vi "Program Device.vi"(0 "Data Cluster In":T1={"Message"="", "Homed?"=FALSE, "NextState"=enum."Timeout", "G.Load"=0.0, "G.Position"=0.0, "Load#"=0, "[G.Loads]"=[], "[TotalLoads]"=[], "[Errors]"=[], "ZeroWait"=0, "Results"=[], "DwellWait"=FALSE, "Test Result"=FALSE, "[CondyleLoads]"=[], "[Max]"=[], "[Min]"=[], "Valid String?"=FALSE, "ScanTime"=timestamp(0 s since 1904-01-01), "ScannedString"="", "LabelDevID"=0, "MfgDate"=timestamp(0 s since 1904-01-01), "[EEPROM Cmds]"=[], "[CalData]"=[], "[A/Ds]"=[], "[A/Dmax]"=[], "[A/Dmin]"=[], "BattMax"=0.0, "BattMin"=0.0, "DwellTime"=2000, "PendingDeviceType"="", "Zero G.load"=0.0, "GAINC Value"="", "Programming Step"=enum."Load EEPROM", "Front Panel Program?"=FALSE, "Final Program?"=FALSE, "PCB Score"=100, "AssyScore"=100, "Pass/Fail #"="", "Result String"="", "Programming Mode"=enum."Initial Program", "Angle Test Step"=enum."Initialize", "Accel Values"=[], "Shutdown Counter"=0, "V1"=0, "V2"=0, "V3"=0, "V4"=0, "EEPROM Data"=[], "Counter"=0, "Page#"=0, "Timer"=timestamp(0 s since 1904-01-01), "Use Mark10?"=FALSE, "Eng-Result#"=0, "DUT Serial #"=0, "Scroll Message?"=FALSE, "Clear Message"=FALSE, "Batt Test Step "=enum."Initialize", "RXTX Window Found?"=FALSE, "Shutdown First Call?"=FALSE, "A2 Delay (msec)"=500, "Support Script"={"Script #"="", "Script Revision"="", "[OEMs]"=[], "[[DeviceTypes]]"=[], "[[DeviceTypesVals]]"=[], "[[List of Errors]]"=[], "Default GAINC"="", "[[ASICtrims]]"=[], "ID For Echo"="", "Condyle A CalFactor"=100, "Condyle B CalFactor"=100, "[OEMs Prefix]"=[], "Packet ID 18"="", "[[Force Table Load Test]]"=[], "[[Force Table AccurTest]]"=[]}, "Serial Table"={"Serial File Path"=path "", "[[Serial Lookup Table]]"=[], "Serial Device Info"=[], "Valid Serial?"=FALSE}, "Target Information"={"Target Brand"="", "Target DeviceType"="", "Target Serial#"=100, "Target Lot#"=0, "Target DevID"=0, "Target Channel"=5}, "Operator"="", "COM Port"="", "Config Path"=path "", "Tx Array"=[], "DUT Parameters"={"Channel"=0, "DeviceID"=0, "Script Rev"=0, "Month"=0, "Day"=0, "Year"=0, "Lot#"=0, "V1"=0, "V2"=0, "V3"=0, "V4"=0, "MFG"=0, "Cal FactorA 10"=0, "Cal FactorB 10  "=0, "Cal FactorA 16"=0, "Cal FactorB 16"=0, "ASICtrim"=[], "TmpChan"=0, "GAINC"="", "Brand"="", "Device"="", "Serial #"=0, "Batt310"=0, "Batt 280"=0}, "FTS Main?"=FALSE, "Loading"={"[Forces]"=[], "[Dwell]"=[], "Loading Step"=enum."Initialize Test"}, "Software Version"="", "Correction Factor"="", "Second Load Test"=FALSE, "Acc Loads"=[], "Mark10 Config"={"H2S%"=[80.0, 85.0, 90.0, 95.0, 100.0], "H2S Speed"=[12.0, 8.0, 6.0, 4.0, 2.0], "H to S"=2.0, "Home Speed"=1.0, "LoadWin"=0.0, "Load Speed"=0.0, "PID"={"Kp"=0.04, "Kd"=0.005001, "Ki"=2.9999999999999923e-05}}, "Channels"={"Transceiver Ch"=5, "Operating Ch"=5, "Start Ch"=0}, "Channel EEPROM"=[], "Load Notes"=[], "Engr Log?"=FALSE, "Time"=[], "Program Retry"=FALSE, "Operator Channel"="", "Target Channel "="", "New Data Program"=FALSE, "NFHU Pass?"=FALSE, "Cycle Number"=0, "Cal Cycle#"=0, "[Avg G.Loads] "=[], "[Avg A/Ds] "=[], "Cal Retry?"=FALSE, "[Total A/Ds]  "=[], "Cycle Num LA"=0, "LA Cycle# "=0, "Shim Num"=0, "Shim#  "=0, "Angle Test?"=FALSE} {"Mark10 Config"."PID"."Ki" min=0.0 max=200.0 format="%.6f"; "Mark10 Config"."PID"."Kd" min=0.0 max=200.0 format="%.6f"; "Mark10 Config"."PID"."Kp" min=0.0 max=200.0 format="%.6f"; "DUT Parameters"."ASICtrim" format="%02x"}, 11 "error in (no error)":errorcluster) -> (4 "Data Cluster Out":T1={"Message"="", "Homed?"=FALSE, "NextState"=enum."Timeout", "G.Load"=0.0, "G.Position"=0.0, "Load#"=0, "[G.Loads]"=[], "[TotalLoads]"=[], "[Errors]"=[], "ZeroWait"=0, "Results"=[], "DwellWait"=FALSE, "Test Result"=FALSE, "[CondyleLoads]"=[], "[Max]"=[], "[Min]"=[], "Valid String?"=FALSE, "ScanTime"=timestamp(0 s since 1904-01-01), "ScannedString"="", "LabelDevID"=0, "MfgDate"=timestamp(0 s since 1904-01-01), "[EEPROM Cmds]"=[], "[CalData]"=[], "[A/Ds]"=[], "[A/Dmax]"=[], "[A/Dmin]"=[], "BattMax"=0.0, "BattMin"=0.0, "DwellTime"=2000, "PendingDeviceType"="", "Zero G.load"=0.0, "GAINC Value"="", "Programming Step"=enum."Load EEPROM", "Front Panel Program?"=FALSE, "Final Program?"=FALSE, "PCB Score"=100, "AssyScore"=100, "Pass/Fail #"="", "Result String"="", "Programming Mode"=enum."Initial Program", "Angle Test Step"=enum."Initialize", "Accel Values"=[], "Shutdown Counter"=0, "V1"=0, "V2"=0, "V3"=0, "V4"=0, "EEPROM Data"=[], "Counter"=0, "Page#"=0, "Timer"=timestamp(0 s since 1904-01-01), "Use Mark10?"=FALSE, "Eng-Result#"=0, "DUT Serial #"=0, "Scroll Message?"=FALSE, "Clear Message"=FALSE, "Batt Test Step "=enum."Initialize", "RXTX Window Found?"=FALSE, "Shutdown First Call?"=FALSE, "A2 Delay (msec)"=500, "Support Script"={"Script #"="", "Script Revision"="", "[OEMs]"=[], "[[DeviceTypes]]"=[], "[[DeviceTypesVals]]"=[], "[[List of Errors]]"=[], "Default GAINC"="", "[[ASICtrims]]"=[], "ID For Echo"="", "Condyle A CalFactor"=100, "Condyle B CalFactor"=100, "[OEMs Prefix]"=[], "Packet ID 18"="", "[[Force Table Load Test]]"=[], "[[Force Table AccurTest]]"=[]}, "Serial Table"={"Serial File Path"=path "", "[[Serial Lookup Table]]"=[], "Serial Device Info"=[], "Valid Serial?"=FALSE}, "Target Information"={"Target Brand"="", "Target DeviceType"="", "Target Serial#"=100, "Target Lot#"=0, "Target DevID"=0, "Target Channel"=5}, "Operator"="", "COM Port"="", "Config Path"=path "", "Tx Array"=[], "DUT Parameters"={"Channel"=0, "DeviceID"=0, "Script Rev"=0, "Month"=0, "Day"=0, "Year"=0, "Lot#"=0, "V1"=0, "V2"=0, "V3"=0, "V4"=0, "MFG"=0, "Cal FactorA 10"=0, "Cal FactorB 10  "=0, "Cal FactorA 16"=0, "Cal FactorB 16"=0, "ASICtrim"=[], "TmpChan"=0, "GAINC"="", "Brand"="", "Device"="", "Serial #"=0, "Batt310"=0, "Batt 280"=0}, "FTS Main?"=FALSE, "Loading"={"[Forces]"=[], "[Dwell]"=[], "Loading Step"=enum."Initialize Test"}, "Software Version"="", "Correction Factor"="", "Second Load Test"=FALSE, "Acc Loads"=[], "Mark10 Config"={"H2S%"=[80.0, 85.0, 90.0, 95.0, 100.0], "H2S Speed"=[12.0, 8.0, 6.0, 4.0, 2.0], "H to S"=2.0, "Home Speed"=1.0, "LoadWin"=0.0, "Load Speed"=0.0, "PID"={"Kp"=0.04, "Kd"=0.005001, "Ki"=2.9999999999999923e-05}}, "Channels"={"Transceiver Ch"=5, "Operating Ch"=5, "Start Ch"=0}, "Channel EEPROM"=[], "Load Notes"=[], "Engr Log?"=FALSE, "Time"=[], "Program Retry"=FALSE, "Operator Channel"="", "Target Channel "="", "New Data Program"=FALSE, "NFHU Pass?"=FALSE, "Cycle Number"=0, "Cal Cycle#"=0, "[Avg G.Loads] "=[], "[Avg A/Ds] "=[], "Cal Retry?"=FALSE, "[Total A/Ds]  "=[], "Cycle Num LA"=0, "LA Cycle# "=0, "Shim Num"=0, "Shim#  "=0, "Angle Test?"=FALSE} {"Mark10 Config"."PID"."Ki" min=0.0 max=200.0 format="%.6f"; "Mark10 Config"."PID"."Kd" min=0.0 max=200.0 format="%.6f"; "Mark10 Config"."PID"."Kp" min=0.0 max=200.0 format="%.6f"; "DUT Parameters"."ASICtrim" format="%02x"}, 6 "Program Successful":bool, 15 "error out":errorcluster)   [LabVIEW 2015]
uses:
  Controls/LocalVars.ctl
  Controls/Gen2 FT states.ctl
  Controls/Iniial Device Programming.ctl
  ProgramStageControl.ctl
  Controls/Batt Cap Steps.ctl
  Controls/Support Script.ctl
  Controls/Serial Table.ctl
  Controls/Device Information.ctl
  Controls/InfoPacket.ctl
  Controls/Loading.ctl
  Controls/Load Step.ctl
  Controls/Mark10 Config.ctl
  Controls/PID parameters.ctl
  Controls/Channels.ctl
  RxTx/XceiverStates.ctl
  RxTx/XceiverCmds.ctl
  Controls/Gen2 FT Globals.vi
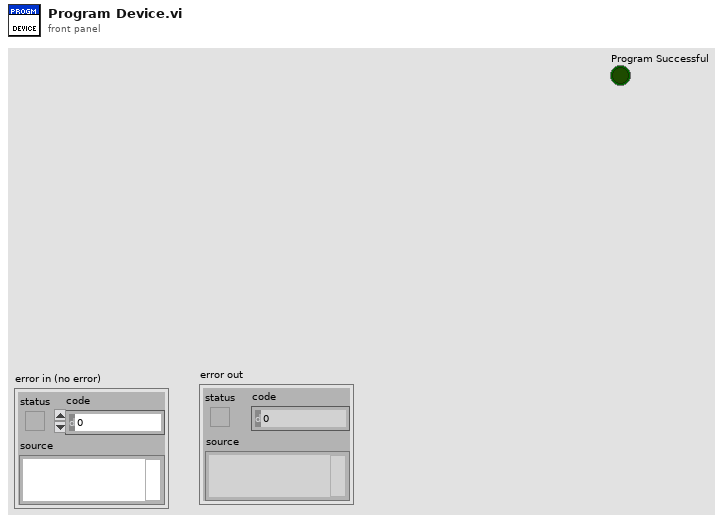
[diagram p1: front panel]
types:
  T1 = typedef "LocalVars.ctl" = cluster{"Message":string, "Homed?":bool, "NextState":T2, "G.Load":dbl, "G.Position":dbl, "Load#":i32, "[G.Loads]":dbl[], "[TotalLoads]":dbl[], "[Errors]":dbl[][], "ZeroWait":u32, "Results":dbl[], "DwellWait":bool, "Test Result":bool, "[CondyleLoads]":dbl[][], "[Max]":dbl[], "[Min]":dbl[], "Valid String?":bool, "ScanTime":timestamp, "ScannedString":string, "LabelDevID":u32, "MfgDate":timestamp, "[EEPROM Cmds]":u8[][], "[CalData]":u8[][], "[A/Ds]":dbl[][], "[A/Dmax]":dbl[], "[A/Dmin]":dbl[], "BattMax":dbl, "BattMin":dbl, "DwellTime":i32, "PendingDeviceType":string, "Zero G.load":dbl, "GAINC Value":string, "Programming Step":T3, "Front Panel Program?":bool, "Final Program?":bool, "PCB Score":i32, "AssyScore":i32, "Pass/Fail #":string, "Result String":string, "Programming Mode":T4, "Angle Test Step":enum16{"Initialize", "Get X", "Get Y", "Get Z", "Next Test"}, "Accel Values":dbl[][], "Shutdown Counter":u32, "V1":i32, "V2":i32, "V3":i32, "V4":i32, "EEPROM Data":i32[][], "Counter":i32, "Page#":i32, "Timer":timestamp, "Use Mark10?":bool, "Eng-Result#":u32, "DUT Serial #":i32, "Scroll Message?":bool, "Clear Message":bool, "Batt Test Step ":T5, "RXTX Window Found?":bool, "Shutdown First Call?":bool, "A2 Delay (msec)":i16, "Support Script":T6, "Serial Table":T7, "Target Information":T8, "Operator":string, "COM Port":string, "Config Path":path, "Tx Array":u8[], "DUT Parameters":T9, "FTS Main?":bool, "Loading":T10, "Software Version":string, "Correction Factor":string, "Second Load Test":bool, "Acc Loads":dbl[][], "Mark10 Config":T12, "Channels":T14, "Channel EEPROM":i32[][], "Load Notes":string[], "Engr Log?":bool, "Time":timestamp[], "Program Retry":bool, "Operator Channel":string, "Target Channel ":string, "New Data Program":bool, "NFHU Pass?":bool, "Cycle Number":i32, "Cal Cycle#":i32, "[Avg G.Loads] ":dbl[], "[Avg A/Ds] ":dbl[][], "Cal Retry?":bool, "[Total A/Ds]  ":dbl[][], "Cycle Num LA":i32, "LA Cycle# ":i32, "Shim Num":i32, "Shim#  ":i32, "Angle Test?":bool}
  T2 = typedef "Gen2 FT states.ctl" = enum16{"---------SETUP-------", "Initialization", "Read Support Data", "Initialize Mark-10", "Initialize Transceiver", "------UTILITIES------", "Change DUT Channel", "Find RxTx Window", "Reset Device", "Scan Channels", "Read Serial Lookup", "Shutdown Device", "ESTOP", "--------USER---------", "Timeout", "-----PROGRAM-----", "Program Device", "------MARK10--------", "Go Home", "MoveUp", "MoveDown", "Goto Load", "Goto Position", "Stop Motor", "---------TESTS--------", "Start Test", "Angle Test", "Load Test", "Load Accuracy Test", "Battery Test", "------RESULTS-------", "End Test", "Display Result", "--------EXIT--------", "Exit"}
  T3 = typedef "Iniial Device Programming.ctl" = enum16{"Load EEPROM", "Send First A1", "Send EEPROM", "Send A1", "Check EEPROM Echo", "Verify transmission", "Programming Successful", "Programming Failed"}
  T4 = typedef "ProgramStageControl.ctl" = enum16{"Initial Program", "GainC", "Scales"}
  T5 = typedef "Batt Cap Steps.ctl" = enum16{"Initialize", "Collect 2.8 Volts", "Collect 3.1 Volts", "Check Results"}
  T6 = typedef "Support Script.ctl" = cluster{"Script #":string, "Script Revision":string, "[OEMs]":string[], "[[DeviceTypes]]":string[][], "[[DeviceTypesVals]]":u16[][], "[[List of Errors]]":string[][], "Default GAINC":string, "[[ASICtrims]]":u8[][], "ID For Echo":string, "Condyle A CalFactor":i32, "Condyle B CalFactor":i32, "[OEMs Prefix]":string[], "Packet ID 18":string, "[[Force Table Load Test]]":dbl[][], "[[Force Table AccurTest]]":dbl[][]}
  T7 = typedef "Serial Table.ctl" = cluster{"Serial File Path":path, "[[Serial Lookup Table]]":string[][], "Serial Device Info":string[], "Valid Serial?":bool}
  T8 = typedef "Device Information.ctl" = cluster{"Target Brand":string, "Target DeviceType":string, "Target Serial#":i32, "Target Lot#":u32, "Target DevID":u32, "Target Channel":u8}
  T9 = typedef "InfoPacket.ctl" = cluster{"Channel":u8, "DeviceID":u32, "Script Rev":u8, "Month":u8, "Day":u8, "Year":u8, "Lot#":u32, "V1":u16, "V2":u16, "V3":u16, "V4":u16, "MFG":u8, "Cal FactorA 10":u8, "Cal FactorB 10  ":u8, "Cal FactorA 16":u8, "Cal FactorB 16":u8, "ASICtrim":u8[], "TmpChan":u8, "GAINC":string, "Brand":string, "Device":string, "Serial #":u64, "Batt310":u16, "Batt 280":u16}
  T10 = typedef "Loading.ctl" = cluster{"[Forces]":dbl[], "[Dwell]":dbl[], "Loading Step":T11}
  T11 = typedef "Load Step.ctl" = enum16{"Initialize Test", "Go Home", "Detect Dev Surface", "Wait to zero Device", "Zero Device", "Do Test", "Test Result"}
  T12 = typedef "Mark10 Config.ctl" = cluster{"H2S%":dbl[], "H2S Speed":dbl[], "H to S":dbl, "Home Speed":dbl, "LoadWin":dbl, "Load Speed":dbl, "PID":T13}
  T13 = typedef "PID parameters.ctl" = cluster{"Kp":dbl, "Kd":dbl, "Ki":dbl}
  T14 = typedef "Channels.ctl" = cluster{"Transceiver Ch":u8, "Operating Ch":u8, "Start Ch":u8}
  T15 = typedef "XceiverStates.ctl" = enum16{"Initialize", "Rx", "Tx", "Raw Mode", "Clear Buffer", "ClearEcho", "Read Buffer", "Close"}
  T16 = typedef "XceiverCmds.ctl" = enum8{"Get Window", "Set Window", "Load&Xmit", "Find Window", "Load CC1101", "Blink LED1", "Blink LED2", "Gen2 Mode", "Request Rev", "Gen2 Mode & Req Rev", "Load Device Settings", "Reset Xceiver", "Set Channel", "Read Channel"}
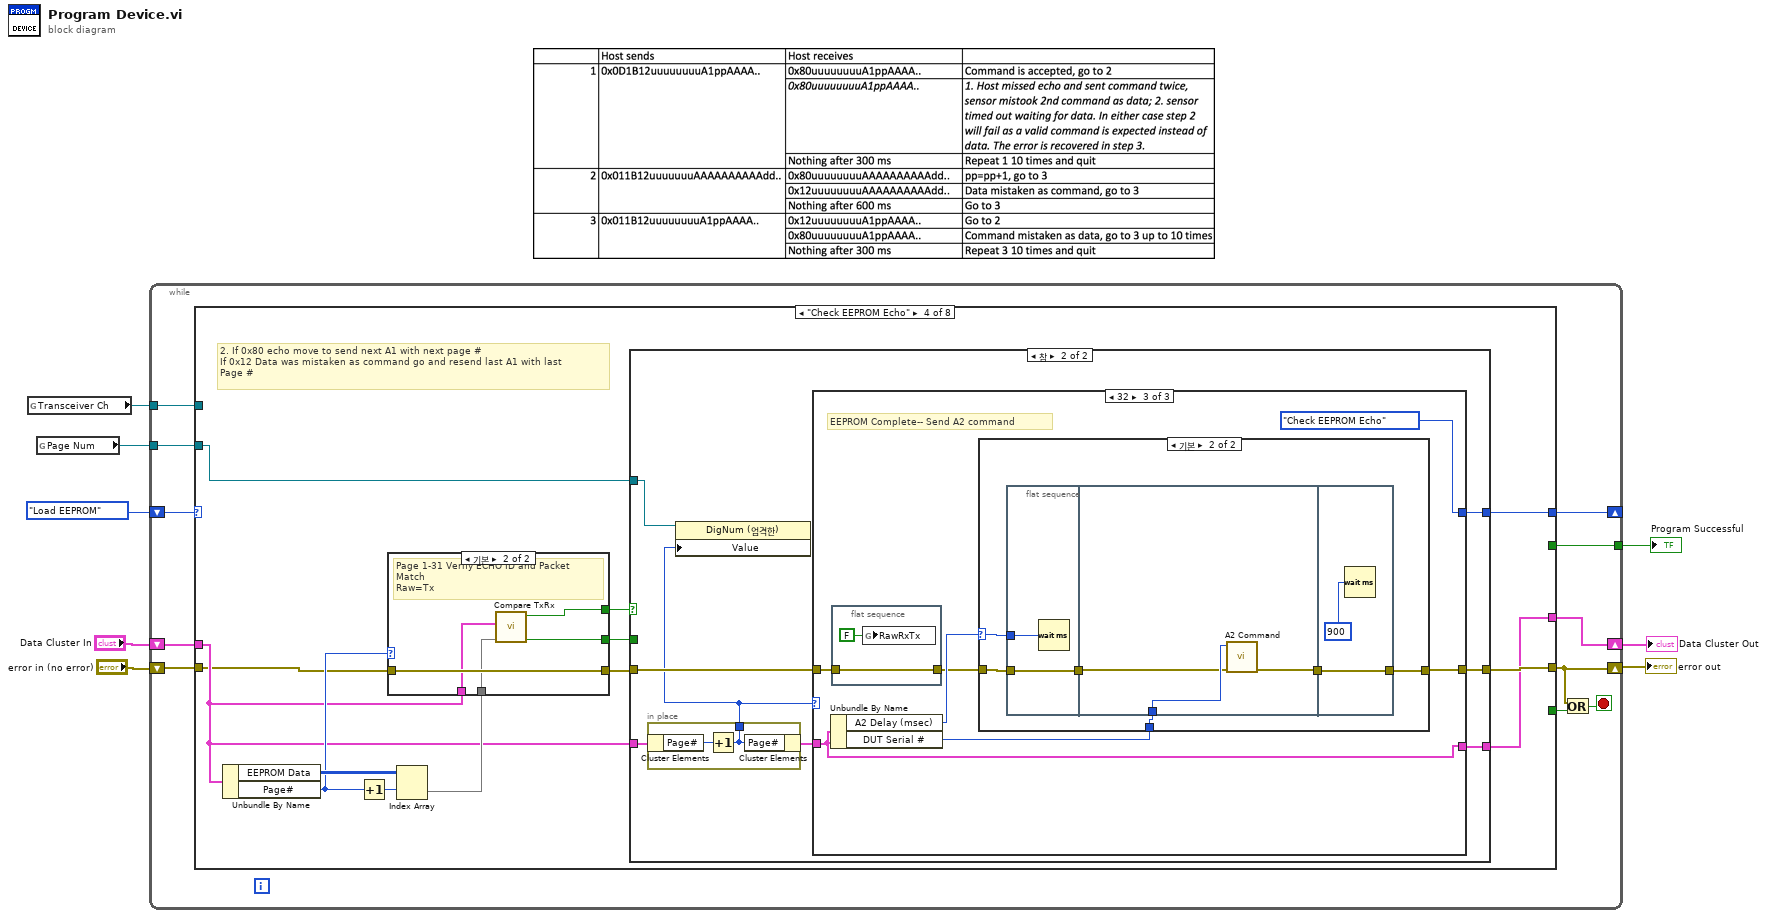
[diagram p0: block diagram]
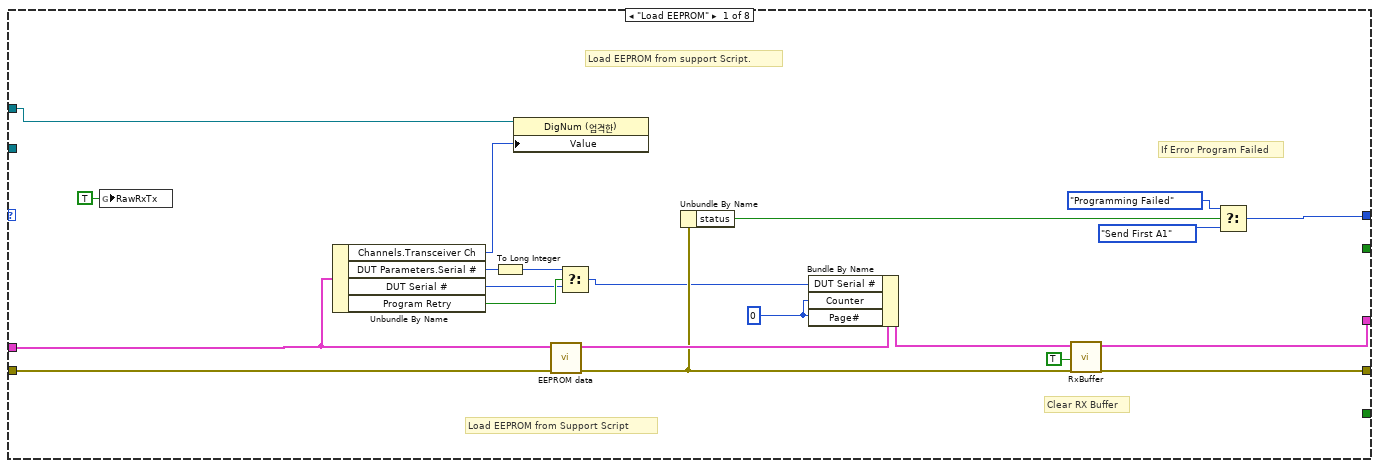
[diagram p2: hidden frame]
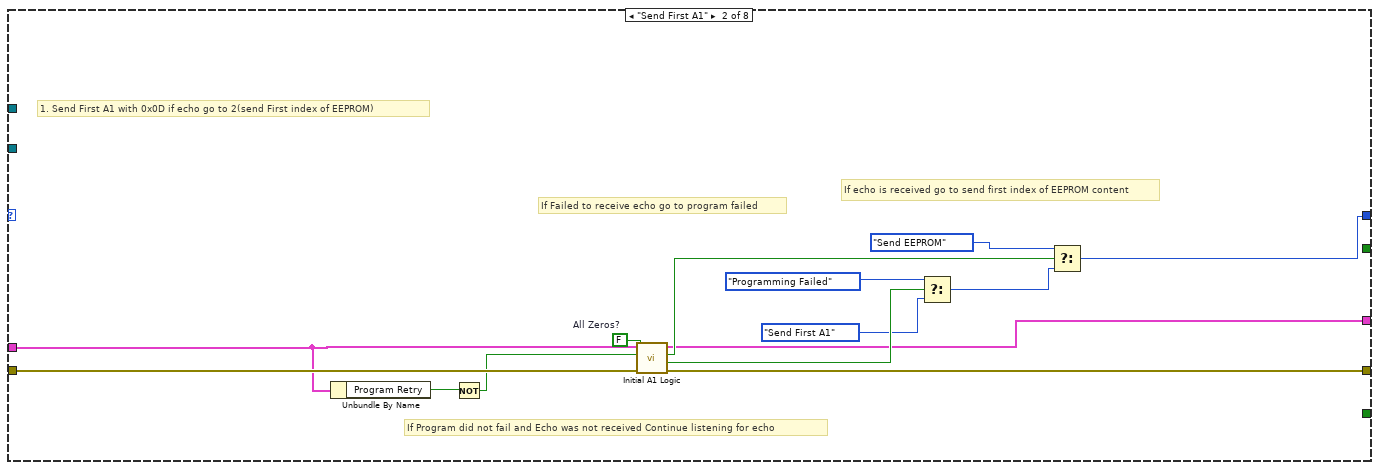
[diagram p3: hidden frame]
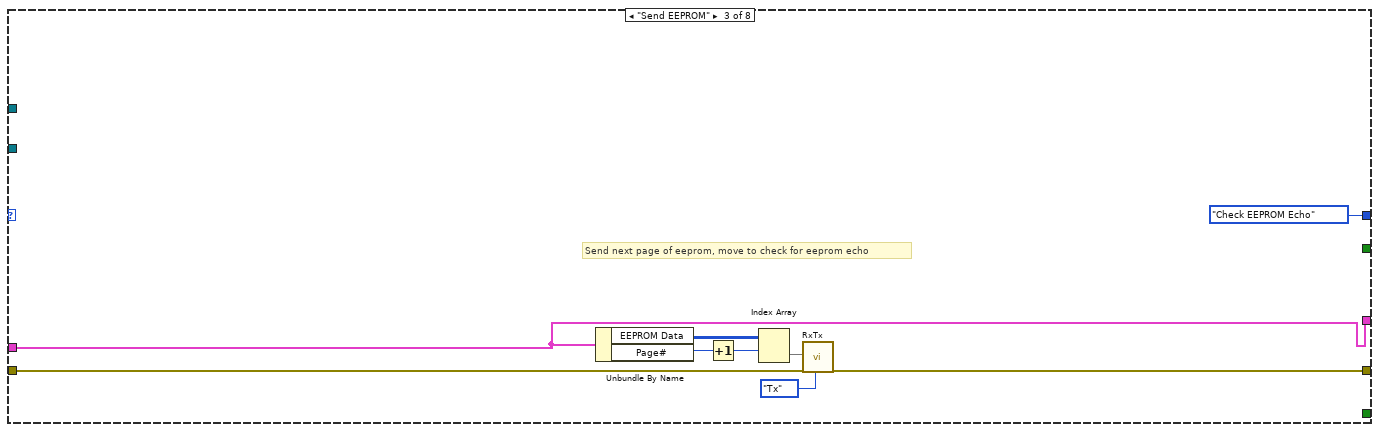
[diagram p4: hidden frame]
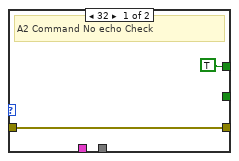
[diagram p5: hidden frame]
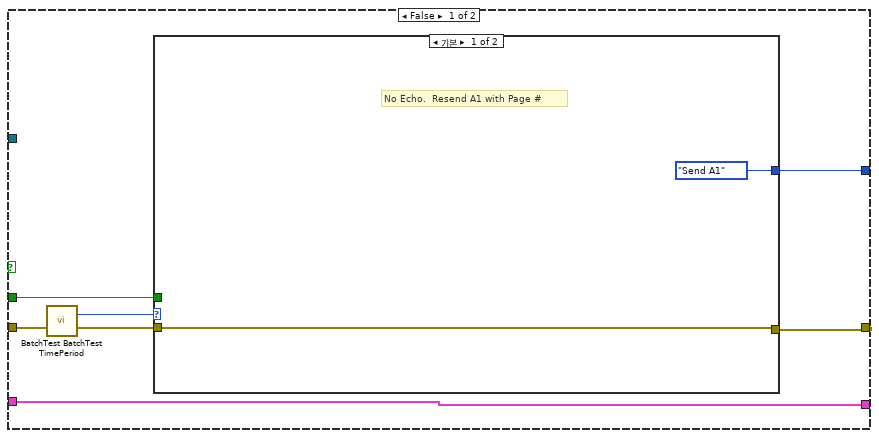
[diagram p6: hidden frame]
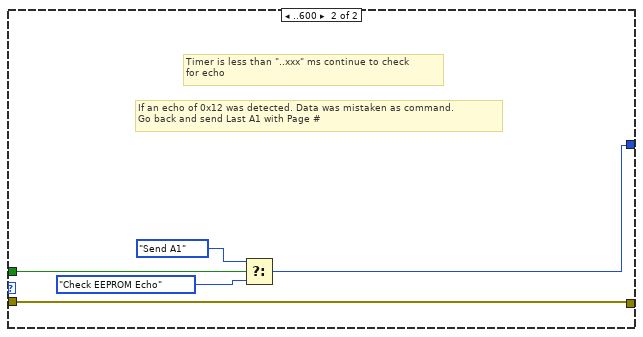
[diagram p7: hidden frame]
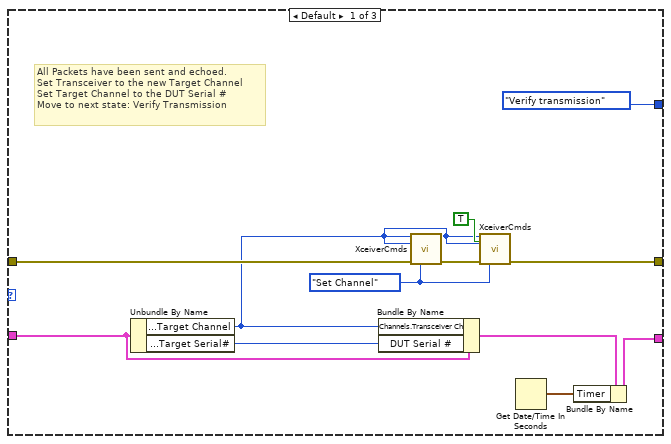
[diagram p8: hidden frame]
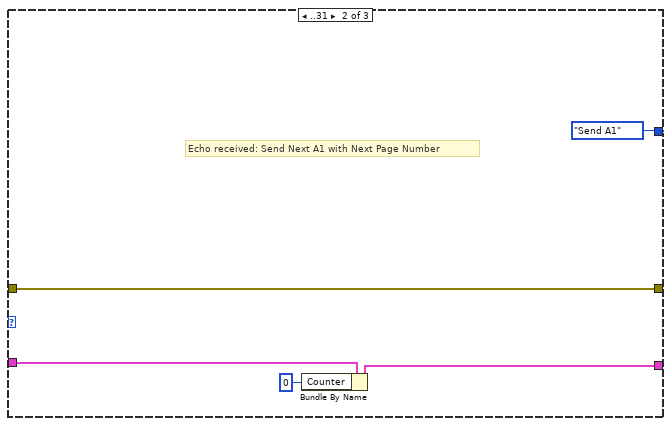
[diagram p9: hidden frame]
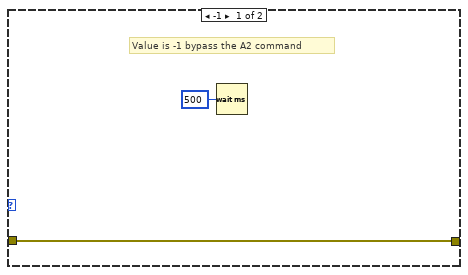
[diagram p10: hidden frame]
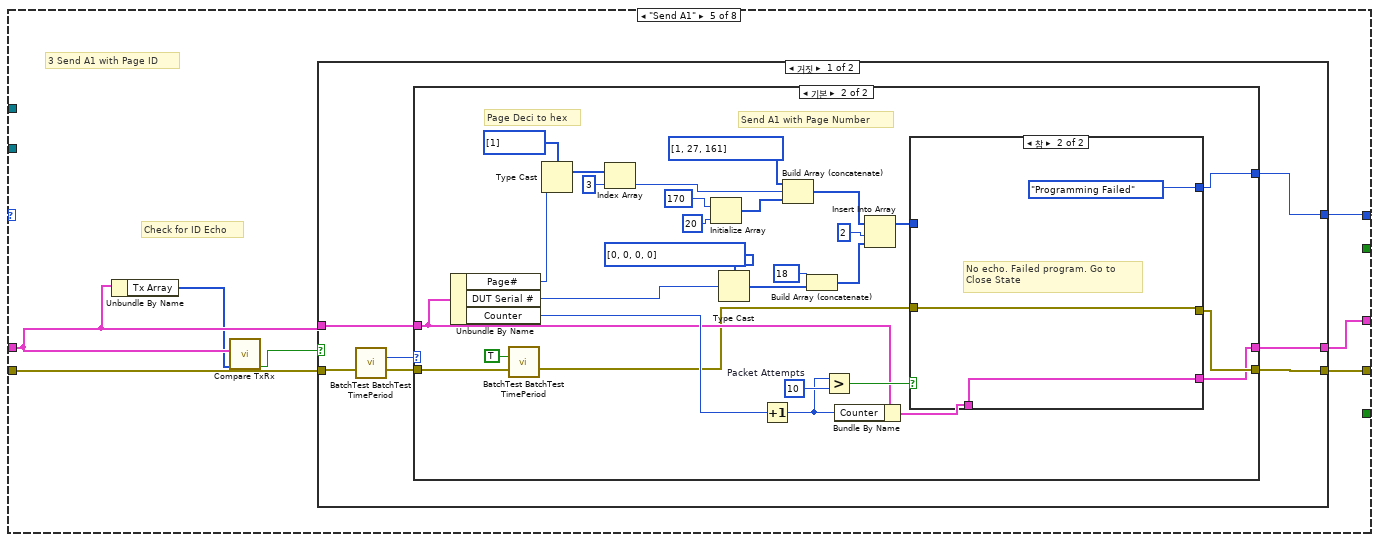
[diagram p11: hidden frame]
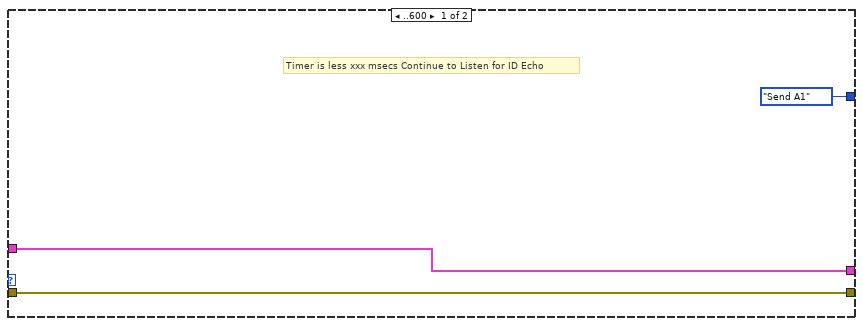
[diagram p12: hidden frame]
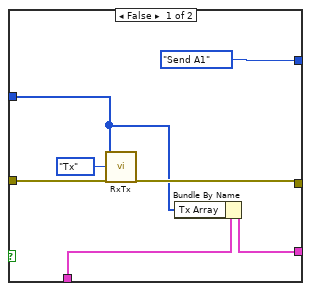
[diagram p13: hidden frame]
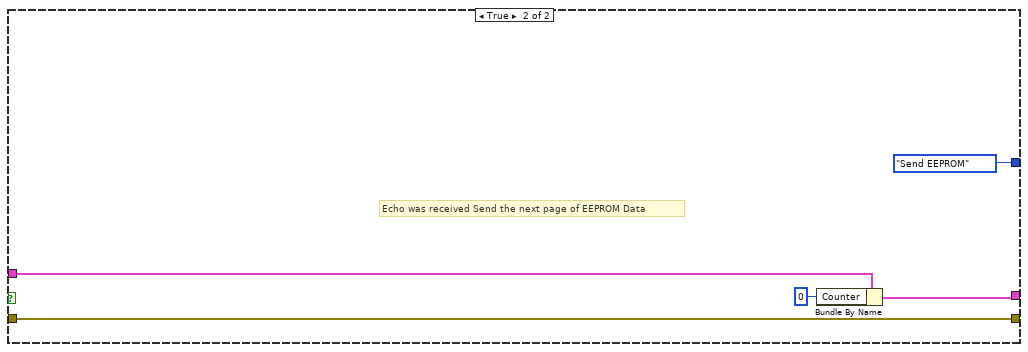
[diagram p14: hidden frame]
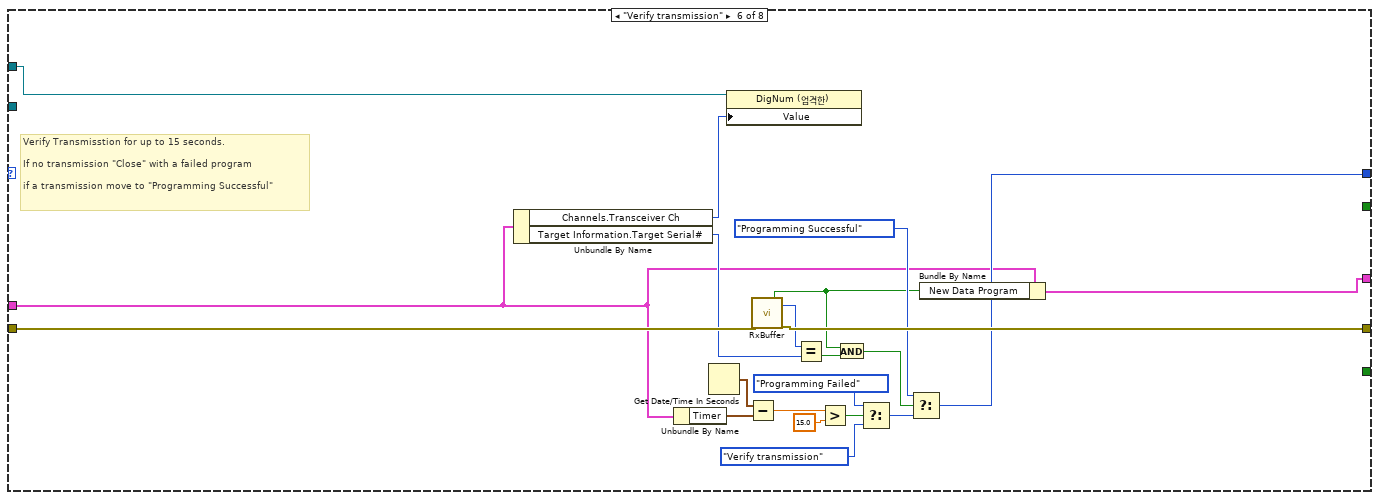
[diagram p15: hidden frame]
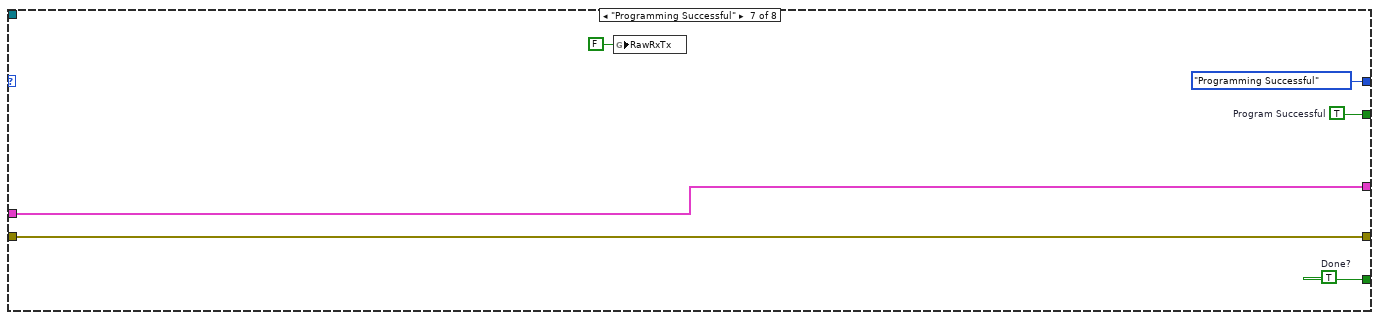
[diagram p16: hidden frame]
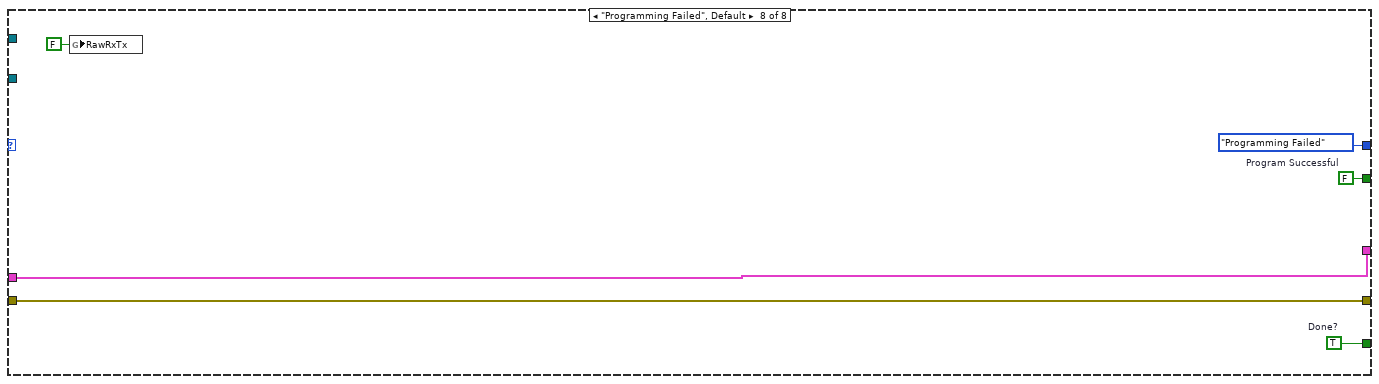
[diagram p17: hidden frame]
diagram:
  n1 = global read "Gen2 FT Globals.vi" "Transceiver Ch"() -> (w1:refnum<vi>)
  n2 = global read "Gen2 FT Globals.vi" "Page Num"() -> (w2:refnum<vi>)
  n3 = while {
    shift-right: [w12] -> w7
    shift-left: "error in (no error)" -> [w19]
    shift-right: [w18] -> _
    shift-left: Iniial_Device_Programming."Load EEPROM" ("t") -> [w15]
    shift-right: [w17] -> w5
    shift-left: "Data Cluster In" -> [w16]
    tunnel: [w13] -> w3
    tunnel: w2 -> [w10]
    tunnel: w1 -> [w9]
    stop <- w14 stop-if-true
    n4 = case shown="\"Check EEPROM Echo\"" w15 {
      tunnel: [w29 w52 w56 w75 w154 w229 w234 w236] -> w12
      tunnel: w19 -> [w33 w53 w57 w64 w148 w228 w234 w236]
      tunnel: [w39 w46 Iniial_Device_Programming."Check EEPROM Echo" ("t") w74 w153 w226 Iniial_Device_Programming."Programming Successful" ("t") Iniial_Device_Programming."Programming Failed" ("t")] -> w18
      tunnel: [_ _ _ _ _ _ w235 w241] -> w11
      tunnel: [w35 w44 w54 w68 w152 w212 w233 w237] -> w17
      tunnel: w16 -> [w27 w42 w54 w65 w150 w213 w233 w237]
      tunnel: [_ _ _ _ _ _ w230 w238] -> w13
      tunnel: w10 -> [_ _ _ w63 _ _ _ _]
      tunnel: w9 -> [w26 _ _ _ _ w210 _ _]
      frame "Load EEPROM" {
        w28 = 0 ("Counter")
        # "Load EEPROM from Support Script"
        # "Load EEPROM from support Script."
        # "If Error Program Failed"
        # "Clear RX Buffer"
        n5 = global write "Gen2 FT Globals.vi" "RawRxTx"(TRUE ("Initialize?")) -> ()
        n6 = Unbundle By Name(w27) -> ("Channels.Transceiver Ch"=w25:u8, "DUT Parameters.Serial #"=w24:u64, "DUT Serial #"=w21:i32, "Program Retry"=w22:bool)
        n7 = To Long Integer(number=w24) -> (32bit integer=w23:i32)
        n8 = property class="DigNum (엄격한)"(reference=w26, "Value"=w25) -> ()  [unwired: 1 in, 2 out]
        n9 = call "EEPROM data.vi"("error in (no error)"=w33, "State-machine Local Variables"=w27) -> ("error out"=w30:errorcluster, "State-machine Local Variables 2"=w34:T1)  [unwired: 8 in]
        n10 = Select(t=w23, s=w22, f=w21) -> (s? t:f=w20:i32)
        n11 = Unbundle By Name(w30) -> ("status"=w38:bool)
        n12 = Bundle By Name(cluster=w34, "DUT Serial #"=w20, "Counter"=w28, "Page#"=w28) -> (w35:T1)
        n13 = call "RxBuffer.vi"("Clear?"=TRUE, "error in (no error)"=w30) -> ("error out"=w29:errorcluster)  [unwired: 6 in, 11 out]
        n14 = Select(t=Iniial_Device_Programming."Programming Failed", s=w38, f=Iniial_Device_Programming."Send First A1") -> (s? t:f=w39:T3)
      }
      frame "Send First A1" {
        w43 = FALSE  # All Zeros?
        # "If Program did not fail and Echo was not received Continue listening for echo"
        # "If Failed to receive echo go to program failed"
        # "If echo is received go to send first index of EEPROM content"
        # "1. Send First A1 with 0x0D if echo go to 2(send First index of EEPROM)"
        n15 = Unbundle By Name(w42) -> ("Program Retry"=w41:bool)
        n16 = Not(x=w41) -> (.not. x?=w40:bool)
        n17 = call "Initial A1 Logic.vi"("error in (no error)"=w53, "All Zeros?"=w43, "0x0D?"=w40, "Data In"=w42) -> ("error out"=w52:errorcluster, "Failed?"=w51:bool, "Echo?"=w45:bool, "Data Out"=w44:T1)  [unwired: 4 in]
        n18 = Select(t=Iniial_Device_Programming."Programming Failed", s=w51, f=Iniial_Device_Programming."Send First A1" ("t")) -> (s? t:f=w48:T3)
        n19 = Select(t=Iniial_Device_Programming."Send EEPROM", s=w45, f=w48) -> (s? t:f=w46:T3)
      }
      frame "Send EEPROM" {
        # "Send next page of eeprom, move to check for eeprom echo"
        n20 = Unbundle By Name(w54) -> ("EEPROM Data"=w62:i32[][], "Page#"=w61:i32)
        n21 = Increment(x=w61) -> (x+1=w58:i32)
        n22 = Index Array(array=w62, index (row)=w58) -> (element=w59:i32[])  [unwired: 1 in]
        n23 = call "RxTx.vi"("[TxData]"=w59, "error in (no error)"=w57, "Action"=XceiverStates."Tx") -> ("error out"=w56:errorcluster)  [unwired: 8 in, 8 out]
      }
      frame "Check EEPROM Echo" {
        # "2. If 0x80 echo move to send next A1 with next page # \nIf 0x12 Data was mistaken as command go and resend last A1 with last\nPage #"
        n24 = Unbundle By Name(w65) -> ("EEPROM Data"=w73:i32[][], "Page#"=w71:i32)
        n25 = Increment(x=w71) -> (x+1=w67:i32)
        n26 = Index Array(array=w73, index (row)=w67) -> (element=w70:i32[])  [unwired: 1 in]
        n27 = case shown="기본" w71 {
          tunnel: [TRUE ("Match?") w80] -> w72
          tunnel: w70 -> [_ w81]
          tunnel: w64 -> [w77 w82]
          tunnel: [w77 w82] -> w69
          tunnel: [_ w78] -> w66
          tunnel: w65 -> [_ w79]
          frame 32 {
            # "A2 Command No echo Check"
          }
          frame Default {
            # "Page 1-31 Verify ECHO ID and Packet Match\nRaw=Tx"
            n28 = call "Compare TxRx.vi"("RawTx"=w81, "Data Cluster In"=w79) -> ("0x12 + Content?"=w78:bool, "0x80 + Content?"=w80:bool)  [unwired: 7 in, 1 out]
          }
        }
        n29 = case shown="참" w72 {
          tunnel: [w87 w102] -> w75
          tunnel: w69 -> [w89 w99]
          tunnel: [w88 w104] -> w74
          tunnel: w65 -> [w84 w103]
          tunnel: [w84 w101] -> w68
          tunnel: w66 -> [w83 _]
          tunnel: w63 -> [_ w98]
          frame False {
            n30 = call "BatchTest BatchTest TimePeriod.vi"("error in (no error)"=w89) -> ("Time(mS)"=w85:u32, "error out"=w86:errorcluster)  [unwired: 13 in]
            n31 = case shown="기본" w85 {
              tunnel: [Iniial_Device_Programming."Send A1" ("t") w93] -> w88
              tunnel: [w90 w96] -> w87
              tunnel: w86 -> [w90 w96]
              tunnel: w83 -> [_ w95]
              frame Default {
                # "No Echo.  Resend A1 with Page #"
              }
              frame ..600 {
                # "If an echo of 0x12 was detected. Data was mistaken as command. \nGo back and send Last A1 with Page #"
                # "Timer is less than \"..xxx\" ms continue to check \nfor echo"
                n32 = Select(t=Iniial_Device_Programming."Send A1", s=w95, f=Iniial_Device_Programming."Check EEPROM Echo" ("t")) -> (s? t:f=w93:T3)
              }
            }
          }
          frame True {
            n33 = in-place {
              in-place-border: [w146] -> w97
              n34 = in-place-cluster #1(w103) -> ("Page#"=w147:i32)
              n35 = Increment(x=w147) -> (x+1=w146:i32)
              n36 = in-place-cluster #1("Page#"=w146) -> (w100:T1)
            }
            n37 = property class="DigNum (엄격한)"(reference=w98, "Value"=w97) -> ()  [unwired: 1 in, 2 out]
            n38 = case shown="32" w97 {
              tunnel: [Iniial_Device_Programming."Verify transmission" ("t") Iniial_Device_Programming."Send A1" ("t") Iniial_Device_Programming."Check EEPROM Echo" ("t")] -> w104
              tunnel: w99 -> [w114 w117 w123]
              tunnel: [w111 w117 w126] -> w102
              tunnel: w100 -> [w115 w121 w127]
              tunnel: [w113 w120 w127] -> w101
              frame Default {
                w109 = TRUE ("RF Chip0 Enable")
                w108 = XceiverCmds."Set Channel" ("XceiverCmd")
                # "All Packets have been sent and echoed.\nSet Transceiver to the new Target Channel\nSet Target Channel to the DUT Serial #\nMove to next state: Verify Transmission"
                n39 = Unbundle By Name(w115) -> ("Target Information.Target Channel"=w105:u8, "Target Information.Target Serial#"=w106:i32)
                n40 = Bundle By Name(cluster=w115, "Channels.Transceiver Ch"=w105, "DUT Serial #"=w106) -> (w110:T1)
                n41 = call "XceiverCmds.vi"("RF Chip0 Channel"=w105, "RF Chip1 Channel"=w105, "error in (no error)"=w114, "XceiverCmd"=w108) -> ("error out"=w107:errorcluster)  [unwired: 9 in, 2 out]
                n42 = call "XceiverCmds.vi"("RF Chip0 Channel"=w105, "RF Chip0 Enable"=w109, "RF Chip1 Enable"=w109, "RF Chip1 Channel"=w105, "error in (no error)"=w107, "XceiverCmd"=w108) -> ("error out"=w111:errorcluster)  [unwired: 7 in, 2 out]
                n43 = Get Date/Time In Seconds() -> (seconds since 1Jan1904=w112:timestamp)
                n44 = Bundle By Name(cluster=w110, "Timer"=w112) -> (w113:T1)
              }
              frame ..31 {
                # "Echo received: Send Next A1 with Next Page Number"
                n45 = Bundle By Name(cluster=w121, "Counter"=0) -> (w120:T1)
              }
              frame 32 {
                # "EEPROM Complete-- Send A2 command"
                n46 = Unbundle By Name(w127) -> ("A2 Delay (msec)"=w124:i16, "DUT Serial #"=w128:i32)
                n47 = flat-sequence {
                  tunnel: w123 -> [w129]
                  tunnel: [w129] -> w122
                  frame #0 {
                    n48 = global write "Gen2 FT Globals.vi" "RawRxTx"(FALSE ("RawRxTx")) -> ()
                  }
                }
                n49 = case shown="기본" w124 {
                  selector: w124 -> [_ w134]
                  tunnel: w122 -> [w131 w137]
                  tunnel: w128 -> [_ w136]
                  tunnel: [w131 w135] -> w126
                  frame -1 {
                    # "Value is -1 bypass the A2 command"
                    n50 = Wait (ms)(milliseconds to wait=u32 500) -> ()  [unwired: 1 out]
                  }
                  frame Default {
                    n51 = flat-sequence {
                      tunnel: w137 -> [w140]
                      tunnel: [w140] -> w138
                      tunnel: w134 -> [w139]
                      tunnel: w138 -> [w142]
                      tunnel: w136 -> [w143]
                      tunnel: [w141] -> w133
                      tunnel: [w145] -> w135
                      tunnel: w133 -> [w145]
                      frame #0 {
                        n52 = Wait (ms)(milliseconds to wait=w139) -> ()  [unwired: 1 out]
                      }
                      frame #1 {
                        n53 = call "A2 Command.vi"("error in (no error)"=w142, "DUT Serial #"=w143) -> ("error out"=w141:errorcluster)  [unwired: 9 in]
                      }
                      frame #2 {
                        n54 = Wait (ms)(milliseconds to wait=u32 900) -> ()  [unwired: 1 out]
                      }
                    }
                  }
                }
              }
            }
          }
        }
      }
      frame "Send A1" {
        # "3 Send A1 with Page ID"
        # "Check for ID Echo"
        n55 = Unbundle By Name(w150) -> ("Tx Array"=w149:u8[])
        n56 = call "Compare TxRx.vi"("RawTx"=w149, "Data Cluster In"=w150) -> ("0x12 + Content?"=w151:bool)  [unwired: 7 in, 2 out]
        n57 = case shown="거짓" w151 {
          tunnel: [w160 w204] -> w154
          tunnel: w148 -> [w161 w204]
          tunnel: [w159 Iniial_Device_Programming."Send EEPROM" ("t")] -> w153
          tunnel: w150 -> [w157 w208]
          tunnel: [w156 w207] -> w152
          frame False {
            n58 = call "BatchTest BatchTest TimePeriod.vi"("error in (no error)"=w161) -> ("Time(mS)"=w155:u32, "error out"=w158:errorcluster)  [unwired: 13 in]
            n59 = case shown="기본" w155 {
              tunnel: w158 -> [w164 w192]
              tunnel: [w164 w177] -> w160
              tunnel: [Iniial_Device_Programming."Send A1" ("t") w176] -> w159
              tunnel: w157 -> [w163 w187]
              tunnel: [w163 w165] -> w156
              frame ..600 {
                # "Timer is less xxx msecs Continue to Listen for ID Echo"
              }
              frame Default {
                w191 = 10  # Packet Attempts
                # "Page Deci to hex"
                # "Send A1 with Page Number"
                n60 = Unbundle By Name(w187) -> ("Page#"=w168:i32, "DUT Serial #"=w175:i32, "Counter"=w190:i32)
                n61 = call "BatchTest BatchTest TimePeriod.vi"("Initialize?"=TRUE, "error in (no error)"=w192) -> ("error out"=w178:errorcluster)  [unwired: 12 in, 1 out]
                n62 = Type Cast(type=u8[] [1], x=w168) -> (*(type *) &x=w170:u8[])
                n63 = Index Array(array=w170, index=3) -> (element=w167:u8)
                n64 = Initialize Array(u8 170, 20 ("dimension size")) -> (w183:u8[])
                n65 = Type Cast(type=u8[] [0, 0, 0, 0] ("initialized array"), x=w175) -> (*(type *) &x=w184:u8[])
                n66 = Increment(x=w190) -> (x+1=w188:i32)
                n67 = Build Array (concatenate)(u8[] [1, 27, 161], w167, w183) -> (w182:u8[])
                n68 = Build Array (concatenate)(u8 18, w184) -> (w180:u8[])
                n69 = Greater?(x=w188, y=w191) -> (0:w189:bool)
                n70 = Bundle By Name(cluster=w187, "Counter"=w188) -> (w166:T1)
                n71 = Insert Into Array(array=w182, index=2, new element=w180) -> (w179:u8[])
                n72 = case shown="참" w189 {
                  tunnel: [Iniial_Device_Programming."Send A1" ("t") Iniial_Device_Programming."Programming Failed" ("t")] -> w176
                  tunnel: w178 -> [w198 w203]
                  tunnel: [w197 w203] -> w177
                  tunnel: w179 -> [w194 _]
                  tunnel: w166 -> [w196 w201]
                  tunnel: [w195 w201] -> w165
                  frame False {
                    n73 = call "RxTx.vi"("[TxData]"=w194, "error in (no error)"=w198, "Action"=XceiverStates."Tx") -> ("error out"=w197:errorcluster)  [unwired: 8 in, 8 out]
                    n74 = Bundle By Name(cluster=w196, "Tx Array"=w194) -> (w195:T1)
                  }
                  frame True {
                    # "No echo. Failed program. Go to \nClose State"
                  }
                }
              }
            }
          }
          frame True {
            # "Echo was received Send the next page of EEPROM Data"
            n75 = Bundle By Name(cluster=w208, "Counter"=0) -> (w207:T1)
          }
        }
      }
      frame "Verify transmission" {
        # "Verify Transmisstion for up to 15 seconds. \n\nIf no transmission \"Close\" with a failed program\n\nif a transmission move to \"Programming Successful\""
        n76 = Unbundle By Name(w213) -> ("Channels.Transceiver Ch"=w209:u8, "Target Information.Target Serial#"=w216:i32)
        n77 = Unbundle By Name(w213) -> ("Timer"=w218:timestamp)
        n78 = Get Date/Time In Seconds() -> (seconds since 1Jan1904=w222:timestamp)
        n79 = property class="DigNum (엄격한)"(reference=w210, "Value"=w209) -> ()  [unwired: 1 in, 2 out]
        n80 = Subtract(x=w222, y=w218) -> (x-y=w220:dbl)
        n81 = call "RxBuffer.vi"("error in (no error)"=w228) -> ("New Data Program"=w211:bool, "DUT Serial Number"=w217:u32, "error out"=w229:errorcluster)  [unwired: 7 in, 9 out]
        n82 = Equal?(x=w217, y=w216) -> (x = y?=w215:bool)
        n83 = Greater?(x=w220, y=15.0) -> (0:w219:bool)
        n84 = And(x=w211, y=w215) -> (x .and. y?=w214:bool)
        n85 = Select(t=Iniial_Device_Programming."Programming Failed", s=w219, f=Iniial_Device_Programming."Verify transmission" ("t")) -> (s? t:f=w224:T3)
        n86 = Select(t=Iniial_Device_Programming."Programming Successful", s=w214, f=w224) -> (s? t:f=w226:T3)
        n87 = Bundle By Name(cluster=w213, "New Data Program"=w211) -> (w212:T1)
      }
      frame "Programming Successful" {
        w230 = TRUE  # Program Successful
        w235 = TRUE  # Done?
        n88 = global write "Gen2 FT Globals.vi" "RawRxTx"(FALSE ("RawRxTx")) -> ()
      }
      frame "Programming Failed", Default {
        w238 = FALSE  # Program Successful
        w241 = TRUE  # Done?
        n89 = global write "Gen2 FT Globals.vi" "RawRxTx"(FALSE ("RawRxTx")) -> ()
      }
    }
    n90 = Or(x=w12, y=w11) -> (x .or. y?=w14:bool)
  }
  "error out" <- w7
  "Data Cluster Out" <- w5
  "Program Successful" <- w3
